vi "Main.vi"() -> ()   [LabVIEW 2017, in "GUI.lvlib"]
doc: "This template is based from the Queued Message Handler design pattern and the Queued Message Handler Project Template that ships with LabVIEW 2014.\n\nThe main difference is that the Queue is private to this module and communication between modules is done via Broadcast and Request events.\n\nRequest events are wrapped via public API methods and are handled in the Event handler loop in this VI.\nAny module can register for Broadcast events sent by this module.\n\nThe Event Handling Loop generates messages based on user interface actions.\n\nThe Message Handling Loop processes messages generated by the Event Handling Loop, or by other messages. The messages are string values, so new messages can be added easily to the Message Cases case structure in the Message Handling Loop. Each message cluster can also provide an optional value for Message Data, which is a variant that can be converted to whatever message-specific data is required.\n_____\nBased on Delacor QMH Project Template 3.1.0.34."
uses:
  GUI.lvlib
  <vilib>/Delacor/Delacor QMH/Libraries/Module Admin_class/Delacor_lib_QMH_Module Admin.lvclass
  Module Buttons--radio button.ctl
  Module Data--cluster.ctl
  Show Panel Argument--cluster.ctl
  Hide Panel Argument--cluster.ctl
  Stop Argument--cluster.ctl
  <vilib>/Delacor/Delacor QMH/Libraries/Module Admin_class/Delacor_lib_QMH_Module Admin.lvclass/Delacor_lib_QMH_Module Admin.ctl
  <vilib>/Delacor/Delacor QMH/Libraries/Module Admin_class/Delacor_lib_QMH_Get External Launch.vi
  <vilib>/Utility/error.llb/Error Cluster From Error Code.vi
  <vilib>/Delacor/Delacor QMH/Libraries/Message Queue_class/Delacor_lib_QMH_Enqueue Message (Single).vi
  <vilib>/ErrorRing/Error Ring.xnode
  <vilib>/Delacor/Delacor QMH/Libraries/Message Queue_class/Delacor_lib_QMH_Message Queue.lvclass
panel:
  in  "Select":T1 caption="Radio Buttons"
  out "Boolean":bool
  in  "Simulate MHL Error":bool
  in  "Simulate EHL Error":bool
  out "error out":errorcluster
  in  "Module Admin":refnum<class "Delacor_lib_QMH_Module Admin.lvclass">
  out "Status":string
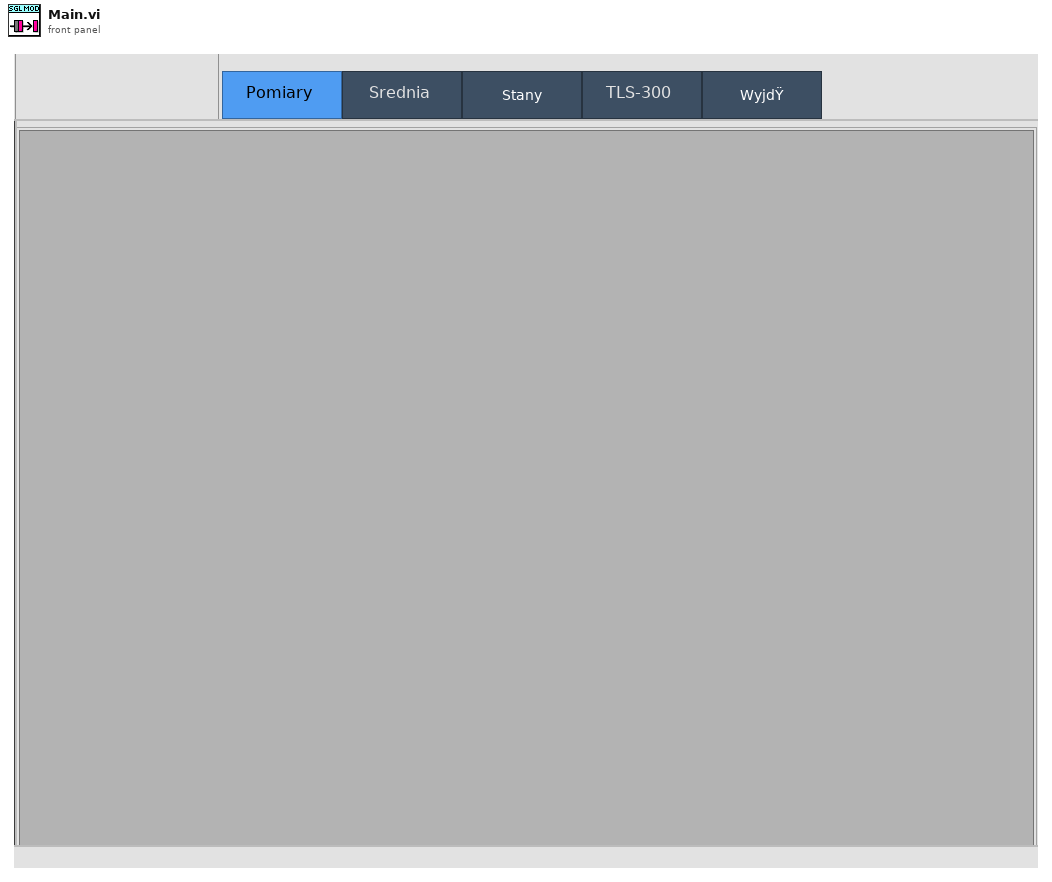
[diagram p1: front panel]
types:
  T1 = typedef "GUI.lvlib/Module Buttons--radio button.ctl" = enum32{"Temperatura", "Srednia", "Stany", "Liczniki", "Exit"}
  T2 = typedef "GUI.lvlib/Request Events--cluster.ctl" = cluster{"Stop Module":refnum<user-event>, "Show Panel":refnum<user-event>, "Hide Panel":refnum<user-event>, "Get Module Execution Status":refnum<user-event>, "Show Diagram":refnum<user-event>}
  T3 = typedef "GUI.lvlib/Module Data--cluster.ctl" = cluster{"Status":string, "subVI Ref.":refnum<vi>[]}
  T4 = typedef "GUI.lvlib/Show Panel Argument--cluster.ctl" = cluster{"Show Panel?":bool}
  T5 = typedef "GUI.lvlib/Hide Panel Argument--cluster.ctl" = cluster{"Hide Panel?":bool}
  T6 = typedef "GUI.lvlib/Stop Argument--cluster.ctl" = cluster{"Origin":string, "Exit via Stop Module Req?":bool, "Wait for Module to stop?":bool}
  T7 = enum32{"Invalid", "Standard", "Closed", "Hidden", "Minimized", "Maximized"}
  T8 = enum32{"invalid lock state", "Not Locked", "Locked (No Password)", "Password-protected"}
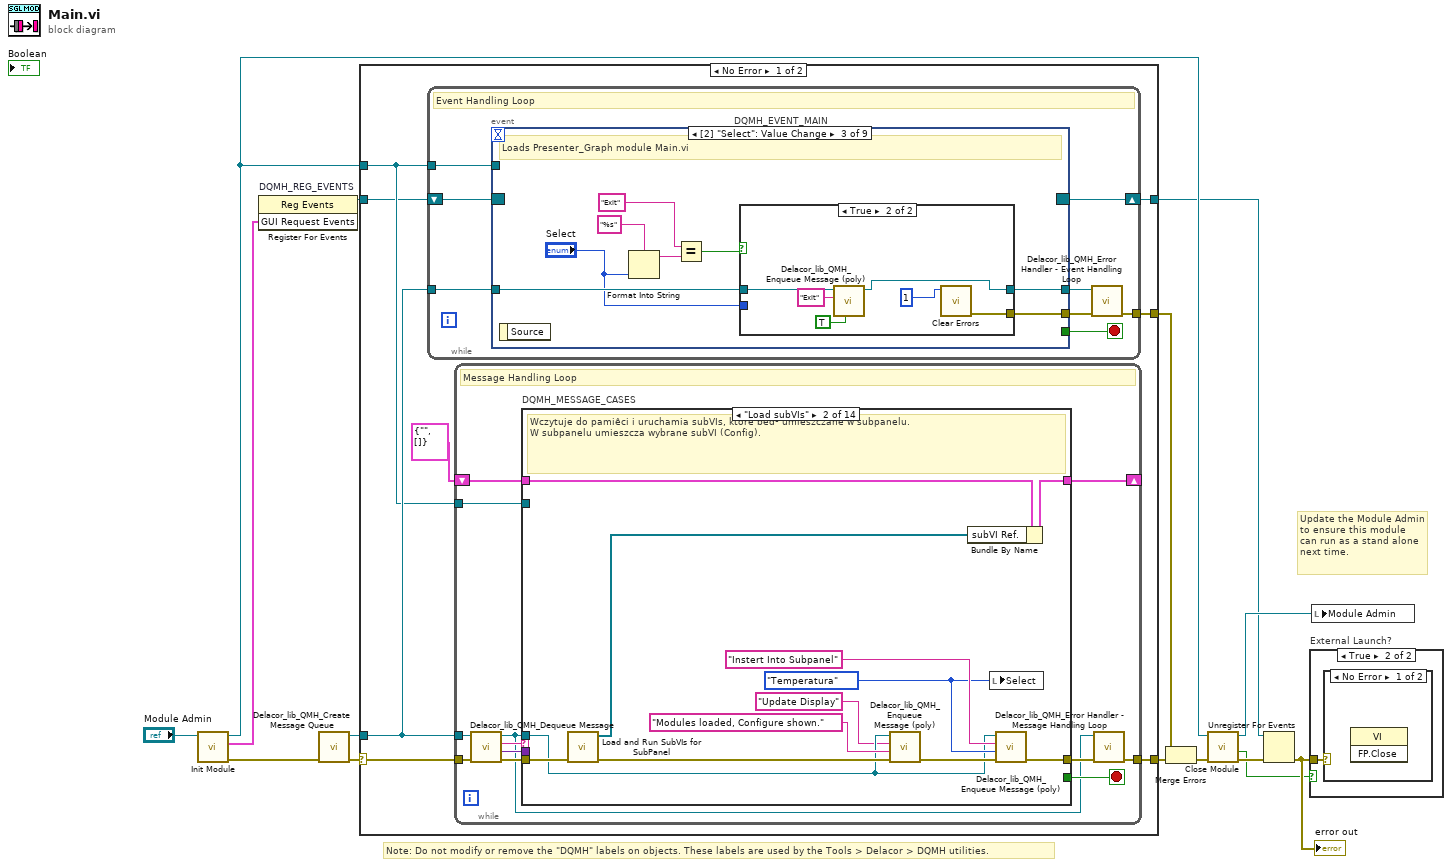
[diagram p0: block diagram]
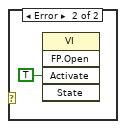
[diagram p3: hidden frame]
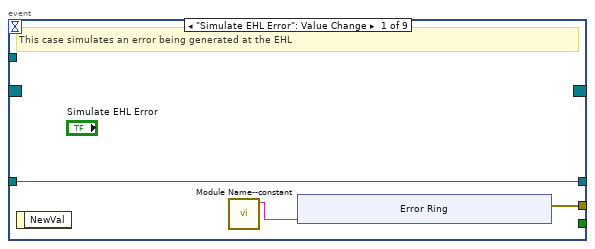
[diagram p4: hidden frame]
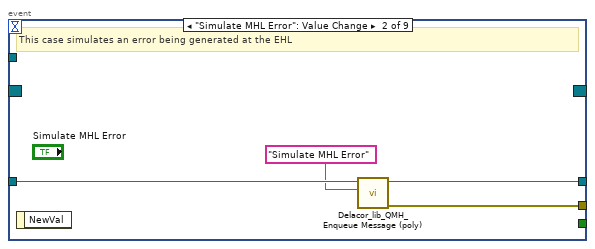
[diagram p5: hidden frame]
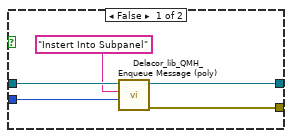
[diagram p6: hidden frame]
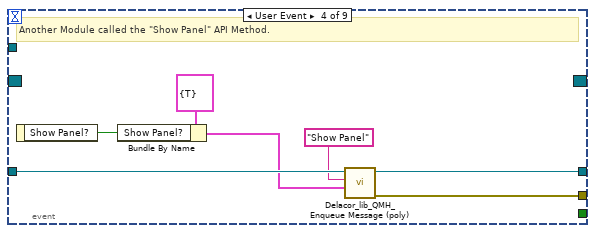
[diagram p7: hidden frame]
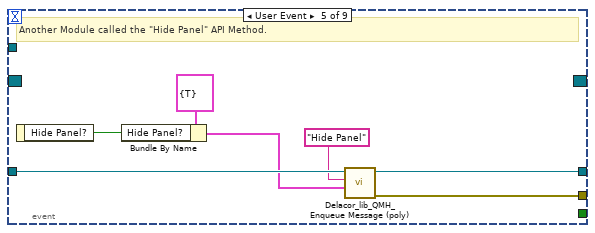
[diagram p8: hidden frame]
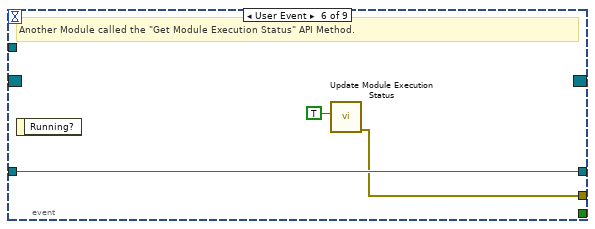
[diagram p9: hidden frame]
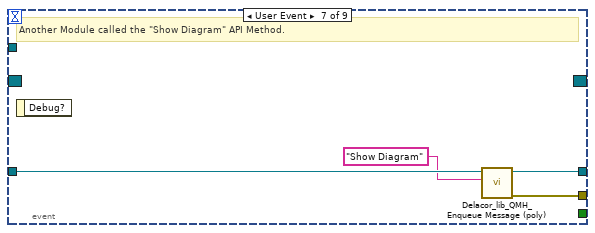
[diagram p10: hidden frame]
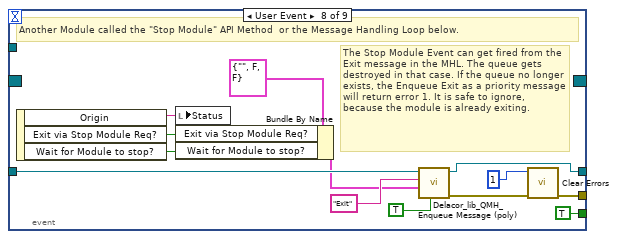
[diagram p11: hidden frame]
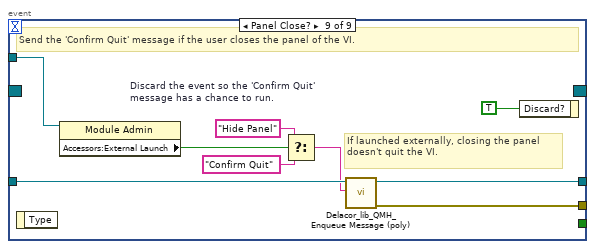
[diagram p12: hidden frame]
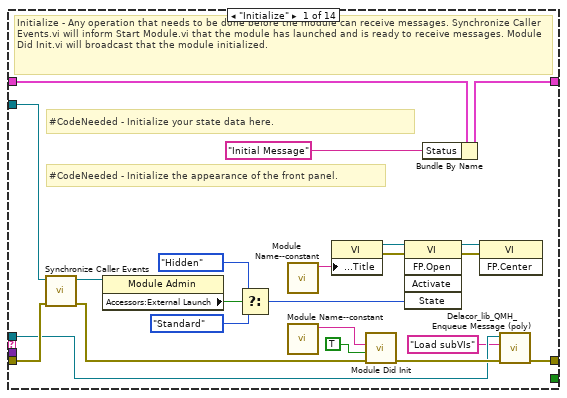
[diagram p13: hidden frame]
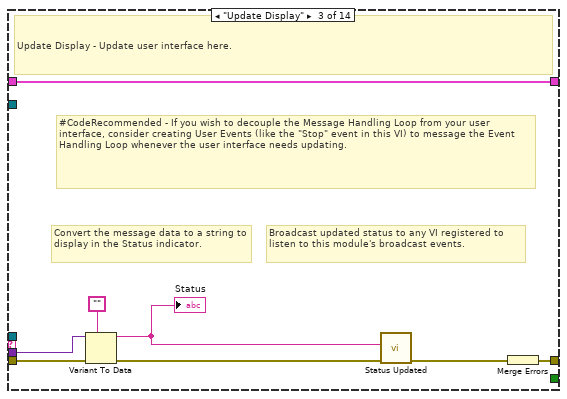
[diagram p14: hidden frame]
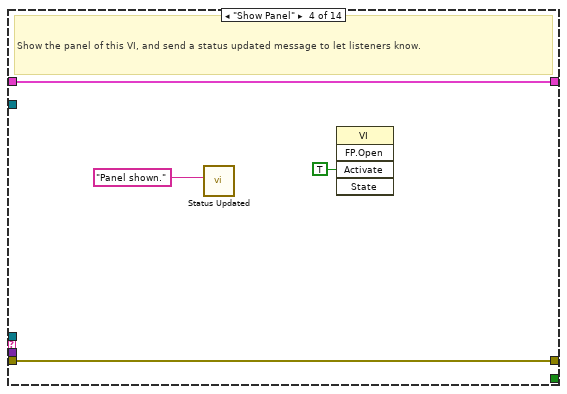
[diagram p15: hidden frame]
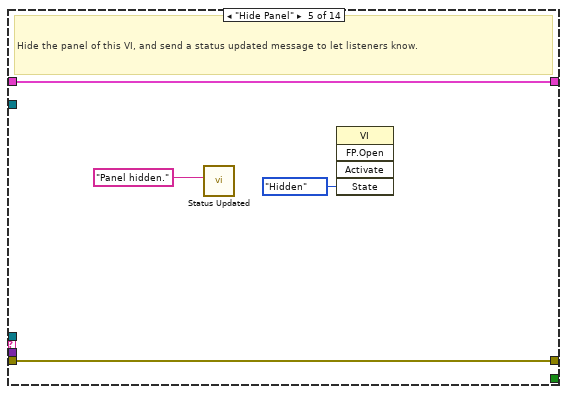
[diagram p16: hidden frame]
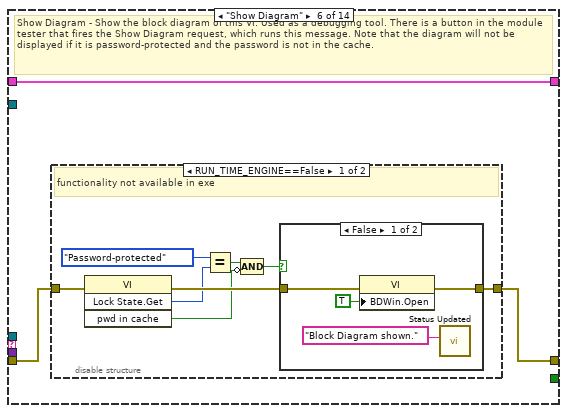
[diagram p17: hidden frame]
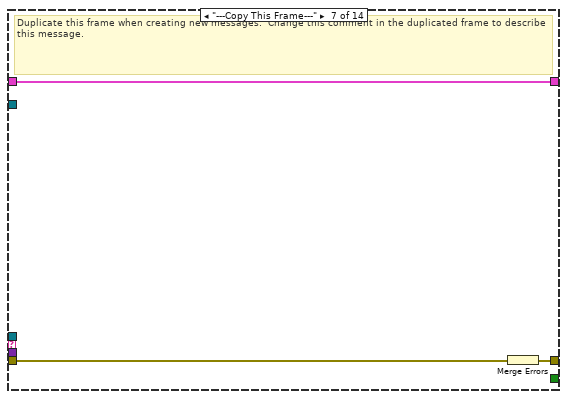
[diagram p20: hidden frame]
diagram:
  # "Note: Do not modify or remove the \"DQMH\" labels on objects. These labels are used by the Tools > Delacor > DQMH utilities."
  # "Update the Module Admin to ensure this module can run as a stand alone next time."
  n1 = call "Init Module.vi"("Singleton Module Admin in"="Module Admin") -> ("error out"=w13:errorcluster, "GUI Request Events"=w11:T2, "Singleton Module Admin out"=w15:refnum<class "Delacor_lib_QMH_Module Admin.lvclass">)  [unwired: 8 in]
  n2 = register-events "DQMH_REG_EVENTS"(w11) -> (reference out=w12:refnum<event-registration>)  [unwired: 2 in, 1 out]
  n3 = call <vilib>:"Delacor_lib_QMH_Create Message Queue.vi"("error in (no error)"=w13) -> ("error out"=w2:errorcluster, "Message Queue"=w10:refnum<class "Delacor_lib_QMH_Message Queue.lvclass">)  [unwired: 9 in]
  n4 = case shown="No Error" w2 {
    selector: w2 -> [w18 w284]
    tunnel: [w23 w284] -> w14
    tunnel: [w22 w289] -> w1
    tunnel: w12 -> [w16 w289]
    tunnel: w10 -> [w20 _]
    tunnel: [w19 _] -> w6
    tunnel: w15 -> [w17 w285]
    frame No Error {
      n5 = while {
        tunnel: w20 -> [w31]
        shift-right: [w29] -> w22
        shift-left: w16 -> [w30]
        tunnel: [w25] -> w19
        tunnel: w17 -> [w24]
        stop <- w27 stop-if-true
        # "Event Handling Loop"
        n6 = event "DQMH_EVENT_MAIN" shown="[2] \"Select\": Value Change" {
          selector: w30 -> [_ _ _ _ _ _ _ _ _]
          dyn-events: [_ _ _ _ _ _ _ _ _] -> w29
          timeout: _ -> [_ _ _ _ _ _ _ _ _]
          tunnel: [_ _ _ _ _ _ _ TRUE ("Discard?") _] -> w27
          tunnel: w31 -> [w34 w45 w53 w71 w78 w81 w85 w96 w106]
          tunnel: [w33 w42 w51 w69 w76 w80 w82 w90 w105] -> w28
          tunnel: [w34 w44 w52 w70 w77 w81 w84 w95 w104] -> w26
          tunnel: w24 -> [_ _ _ _ _ _ _ _ w100]
          event "Simulate EHL Error": Value Change {
            # "This case simulates an error being generated at the EHL"
            n7 = event-data() -> ()  [unwired: 1 in, 1 out]
            n8 = call "Module Name--constant.vi"() -> ("Module Name"=w32:string)  [unwired: 11 in]
            n9 = xnode "Error Ring"("parameter 0"=w32) -> ("error out"=w33:errorcluster)
          }
          event "Simulate MHL Error": Value Change {
            # "This case simulates an error being generated at the EHL"
            n10 = event-data() -> ()  [unwired: 1 in, 1 out]
            n11 = call-poly <vilib>:"Delacor_lib_QMH_Enqueue Message (poly).vi"("Message"="Simulate MHL Error", "Message Queue in"=w45) -> ("error out"=w42:errorcluster, "Message Queue out"=w44:refnum<class "Delacor_lib_QMH_Message Queue.lvclass">)  [unwired: 8 in]
          }
          event Value Change {
            # "Loads Presenter_Graph module Main.vi"
            n12 = event-data() -> ()  [unwired: 1 in, 1 out]
            n13 = Format Into String(format string="%s", "Select") -> (resulting string=w49:string)  [unwired: 2 in, 1 out]
            n14 = Equal?(x="Exit", y=w49) -> (x = y?=w47:bool)
            n15 = case shown="True" w47 {
              tunnel: w53 -> [w58 w61]
              tunnel: [w57 w60] -> w52
              tunnel: [w56 w64] -> w51
              tunnel: "Select" -> [w54 _]
              frame False {
                n16 = call-poly <vilib>:"Delacor_lib_QMH_Enqueue Message (poly).vi"("Message Data"=w54, "Message"="Instert Into Subpanel", "Message Queue in"=w58) -> ("error out"=w56:errorcluster, "Message Queue out"=w57:refnum<class "Delacor_lib_QMH_Message Queue.lvclass">)  [unwired: 7 in]
              }
              frame True {
                n17 = call-poly <vilib>:"Delacor_lib_QMH_Enqueue Message (poly).vi"("Priority Message? (F)"=TRUE, "Message"="Exit", "Message Queue in"=w61) -> ("Message Queue out"=w60:refnum<class "Delacor_lib_QMH_Message Queue.lvclass">)  [unwired: 7 in, 1 out]
                n18 = call <vilib>:"Clear Errors.vi"("specific error code to clear (0: all)"=1) -> ("error out"=w64:errorcluster)  [unwired: 5 in, 1 out]
              }
            }
          }
          event User Event {
            # "Another Module called the \"Show Panel\" API Method."
            n19 = event-data() -> ("Show Panel?"=w67:bool)  [unwired: 1 in]
            n20 = Bundle By Name(cluster=T4 {"Show Panel?"=TRUE} ("Show Panel Argument"), "Show Panel?"=w67) -> (w65:T4)
            n21 = call-poly <vilib>:"Delacor_lib_QMH_Enqueue Message (poly).vi"("Message Data"=w65, "Message"="Show Panel", "Message Queue in"=w71) -> ("error out"=w69:errorcluster, "Message Queue out"=w70:refnum<class "Delacor_lib_QMH_Message Queue.lvclass">)  [unwired: 7 in]
          }
          event User Event {
            # "Another Module called the \"Hide Panel\" API Method."
            n22 = event-data() -> ("Hide Panel?"=w73:bool)  [unwired: 1 in]
            n23 = Bundle By Name(cluster=T5 {"Hide Panel?"=TRUE} ("Hide Panel Argument"), "Hide Panel?"=w73) -> (w72:T5)
            n24 = call-poly <vilib>:"Delacor_lib_QMH_Enqueue Message (poly).vi"("Message Data"=w72, "Message"="Hide Panel", "Message Queue in"=w78) -> ("error out"=w76:errorcluster, "Message Queue out"=w77:refnum<class "Delacor_lib_QMH_Message Queue.lvclass">)  [unwired: 7 in]
          }
          event User Event {
            # "Another Module called the \"Get Module Execution Status\" API Method."
            n25 = event-data() -> ()  [unwired: 1 in, 1 out]
            n26 = call "Update Module Execution Status.vi"("Running?"=TRUE) -> ("error out"=w80:errorcluster)  [unwired: 10 in]
          }
          event User Event {
            # "Another Module called the \"Show Diagram\" API Method."
            n27 = event-data() -> ()  [unwired: 1 in, 1 out]
            n28 = call-poly <vilib>:"Delacor_lib_QMH_Enqueue Message (poly).vi"("Message"="Show Diagram", "Message Queue in"=w85) -> ("error out"=w82:errorcluster, "Message Queue out"=w84:refnum<class "Delacor_lib_QMH_Message Queue.lvclass">)  [unwired: 8 in]
          }
          event User Event {
            # "The Stop Module Event can get fired from the Exit message in the MHL. The queue gets destroyed in that case. If the queue no longer exists, the Enqueue Exit as a priority message will return error 1. It is safe to ignore, because the module is already exiting."
            # "Another Module called the \"Stop Module\" API Method  or the Message Handling Loop below."
            n29 = event-data() -> ("Origin"=w94:string, "Exit via Stop Module Req?"=w88:bool, "Wait for Module to stop?"=w87:bool)  [unwired: 1 in]
            n30 = local write "Status"(w94) -> ()
            n31 = Bundle By Name(cluster=T6 {"Origin"="", "Exit via Stop Module Req?"=FALSE, "Wait for Module to stop?"=FALSE} ("Stop Argument"), "Exit via Stop Module Req?"=w88, "Wait for Module to stop?"=w87) -> (w86:T6)
            n32 = call-poly <vilib>:"Delacor_lib_QMH_Enqueue Message (poly).vi"("Priority Message? (F)"=TRUE, "Message Data"=w86, "Message"="Exit", "Message Queue in"=w96) -> ("error out"=w91:errorcluster, "Message Queue out"=w95:refnum<class "Delacor_lib_QMH_Message Queue.lvclass">)  [unwired: 6 in]
            n33 = call <vilib>:"Clear Errors.vi"("error in (no error)"=w91, "specific error code to clear (0: all)"=1) -> ("error out"=w90:errorcluster)  [unwired: 4 in, 1 out]
          }
          event Panel Close? {
            w107 = TRUE  # Discard the event so the 'Confirm Quit' message has a chance to run.
            # "If launched externally, closing the panel doesn't quit the VI."
            # "Send the 'Confirm Quit' message if the user closes the panel of the VI."
            n34 = event-data() -> ()  [unwired: 1 in, 1 out]
            n35 = property class="Module Admin"(reference=w100) -> ("Accessors:External Launch"=w99:bool)  [unwired: 1 in, 2 out]
            n36 = Select(t="Hide Panel" ("Message"), s=w99, f="Confirm Quit" ("Message")) -> (s? t:f=w101:string)
            n37 = call-poly <vilib>:"Delacor_lib_QMH_Enqueue Message (poly).vi"("Message"=w101, "Message Queue in"=w106) -> ("error out"=w105:errorcluster, "Message Queue out"=w104:refnum<class "Delacor_lib_QMH_Message Queue.lvclass">)  [unwired: 8 in]
            n38 = event-data("Discard?"=w107) -> ()  [unwired: 1 in, 1 out]
          }
        }
        n39 = call-dynamic "Delacor_lib_QMH_Error Handler - Event Handling Loop.vi"("error in (no error)"=w28, "Message Queue in"=w26) -> ("dup error in"=w25:errorcluster)  [unwired: 8 in, 1 out]
      }
      n40 = while {
        tunnel: w20 -> [w111]
        shift-right: [w117] -> _
        shift-left: T3 {"Status"="", "subVI Ref."=[]} ("Data Cluster") -> [w118]
        tunnel: w18 -> [w115]
        tunnel: [w109] -> w23
        tunnel: w17 -> [w108]
        stop <- w116 stop-if-true
        # "Message Handling Loop"
        n41 = call-dynamic "Delacor_lib_QMH_Dequeue Message.vi"("error in (no error)"=w115, "Message Queue in"=w111) -> ("error out"=w114:errorcluster, "Message Data"=w112:variant, "Message"=w113:string, "Message Queue out"=w110:refnum<class "Delacor_lib_QMH_Message Queue.lvclass">)  [unwired: 6 in]
        n42 = case "DQMH_MESSAGE_CASES" shown="\"Load subVIs\"" w113 {
          selector: w113 -> [_ _ _ _ _ _ _ _ _ _ _ _ _ w271]
          tunnel: w110 -> [w121 w143 _ _ _ _ _ w191 _ _ w227 w242 w262 _]
          tunnel: w114 -> [w131 w150 w159 w165 w166 w171 w189 w207 w211 w216 w233 w246 w264 _]
          tunnel: [w122 w148 w160 w165 w166 w170 w187 w208 w209 w214 w224 w244 w259 w272] -> w119
          tunnel: w118 -> [w130 w153 w161 w164 w169 w172 w188 w202 w210 w215 w232 w245 w251 w273]
          tunnel: [w129 w152 w161 w164 w169 w172 w188 w202 w210 w215 w232 w245 w251 w273] -> w117
          tunnel: [_ _ _ _ _ _ _ _ _ _ _ _ w261 _] -> w116
          tunnel: w112 -> [_ _ w158 _ _ _ _ w205 _ _ w231 _ w258 _]
          tunnel: w108 -> [w132 _ _ _ _ _ _ _ _ _ w226 _ w252 _]
          frame "Initialize" {
            # "#CodeNeeded - Initialize the appearance of the front panel."
            # "#CodeNeeded - Initialize your state data here."
            # "Initialize - Any operation that needs to be done before the module can receive messages. Synchronize Caller Events.vi will inform Start Module.vi that the module has launched and is ready to receive messages. Module Did Init.vi will broadcast that the module initialized."
            n43 = call "Synchronize Caller Events.vi"("error in (no error)"=w131, "Singleton Module Admin in"=w132) -> ("error out"=w125:errorcluster, "Singleton Module Admin out"=w124:refnum<class "Delacor_lib_QMH_Module Admin.lvclass">)  [unwired: 8 in]
            n44 = property class="Module Admin"(reference=w124) -> ("Accessors:External Launch"=w136:bool)  [unwired: 1 in, 2 out]
            n45 = Select(t=T7."Hidden" ("State"), s=w136, f=T7."Standard" ("State")) -> (s? t:f=w133:T7)
            n46 = call "Module Name--constant.vi"() -> ("Module Name"=w141:string)  [unwired: 11 in]
            n47 = call "Module Name--constant.vi"() -> ("Module Name"=w126:string)  [unwired: 11 in]
            n48 = property class="VI"("Front Panel.Title"=w141) -> (reference out=w139:refnum<vi>, error out=w140:errorcluster)  [unwired: 2 in]
            n49 = call "Module Did Init.vi"("error in (no error)"=w125, "Initialized?"=TRUE, "Origin"=w126) -> ("error out"=w123:errorcluster)  [unwired: 8 in]
            n50 = invoke class="VI" method="FP.Open"(reference=w139, error in=w140, "State"=w133) -> (reference out=w138:refnum<vi>, error out=w137:errorcluster)  [unwired: 2 in, 3 out]
            n51 = Bundle By Name(cluster=w130, "Status"="Initial Message" ("Initial Message")) -> (w129:T3)
            n52 = invoke class="VI" method="FP.Center"(reference=w138, error in=w137) -> ()  [unwired: 1 in, 3 out]
            n53 = call-poly <vilib>:"Delacor_lib_QMH_Enqueue Message (poly).vi"("error in (no error)"=w123, "Message"="Load subVIs", "Message Queue in"=w121) -> ("error out"=w122:errorcluster)  [unwired: 7 in, 1 out]
          }
          frame "Load subVIs" {
            w147 = Module_Buttons--radio_button."Temperatura" ("Select")
            # "Wczytuje do pamiêci i uruchamia subVIs, które bêd¹ umieszczane w subpanelu.\nW subpanelu umieszcza wybrane subVI (Config)."
            n54 = call "Load and Run SubVIs for SubPanel.vi"("error in (no error)"=w150) -> ("error out"=w146:errorcluster, "subVIs Ref."=w151:refnum<vi>[])  [unwired: 9 in]
            n55 = call-poly <vilib>:"Delacor_lib_QMH_Enqueue Message (poly).vi"("error in (no error)"=w146, "Message Data"="Modules loaded, Configure shown." ("Message"), "Message"="Update Display", "Message Queue in"=w143) -> ("error out"=w145:errorcluster)  [unwired: 6 in, 1 out]
            n56 = Bundle By Name(cluster=w153, "subVI Ref."=w151) -> (w152:T3)
            n57 = local write "Select"(w147) -> ()
            n58 = call-poly <vilib>:"Delacor_lib_QMH_Enqueue Message (poly).vi"("error in (no error)"=w145, "Message Data"=w147, "Message"="Instert Into Subpanel", "Message Queue in"=w143) -> ("error out"=w148:errorcluster)  [unwired: 6 in, 1 out]
          }
          frame "Update Display" {
            # "Broadcast updated status to any VI registered to listen to this module's broadcast events."
            # "Convert the message data to a string to display in the Status indicator."
            # "#CodeRecommended - If you wish to decouple the Message Handling Loop from your user interface, consider creating User Events (like the \"Stop\" event in this VI) to message the Event Handling Loop whenever the user interface needs updating."
            # "Update Display - Update user interface here."
            n59 = Variant To Data(error in=w159, type="", Variant=w158) -> (data=w156:string, error out=w155:errorcluster)
            "Status" <- w156
            n60 = call "Status Updated.vi"("error in (no error)"=w155, "Status"=w156) -> ("error out"=w154:errorcluster)  [unwired: 9 in]
            n61 = Merge Errors(w154) -> (w160:errorcluster)
          }
          frame "Show Panel" {
            # "Show the panel of this VI, and send a status updated message to let listeners know."
            n62 = call "Status Updated.vi"("Status"="Panel shown." ("format string")) -> ()  [unwired: 10 in, 1 out]
            n63 = invoke class="VI" method="FP.Open"("Activate"=TRUE ("Activate?")) -> ()  [unwired: 4 in, 5 out]
          }
          frame "Hide Panel" {
            # "Hide the panel of this VI, and send a status updated message to let listeners know."
            n64 = call "Status Updated.vi"("Status"="Panel hidden." ("format string")) -> ()  [unwired: 10 in, 1 out]
            n65 = invoke class="VI" method="FP.Open"("State"=T7."Hidden") -> ()  [unwired: 4 in, 5 out]
          }
          frame "Show Diagram" {
            # "Show Diagram - Show the block diagram of this VI. Used as a debugging tool. There is a button in the module tester that fires the Show Diagram request, which runs this message. Note that the diagram will not be displayed if it is password-protected and the password is not in the cache."
            n66 = disable-structure shown="RUN_TIME_ENGINE==False" {
              disable-tunnel: [w180 w186] -> w170
              disable-tunnel: w171 -> [w179 w186]
              frame condition #0 (active) {
                # "functionality not available in exe"
                n67 = invoke class="VI" method="Lock State.Get"(error in=w179) -> (error out=w178:errorcluster, "Get Lock State"=w177:T8, "pwd in cache"=w174:bool)  [unwired: 3 in, 1 out]
                n68 = Equal?(x=T8."Password-protected", y=w177) -> (x = y?=w175:bool)
                n69 = Compound Arithmetic op=AND(w175, invert w174) -> (w173:bool)
                n70 = case shown="False" w173 {
                  tunnel: [w183 w185] -> w180
                  tunnel: w178 -> [w181 w185]
                  frame False {
                    n71 = property class="VI"(error in=w181, "BDWin.Open"=TRUE ("Block Diagram Window:Open")) -> (error out=w183:errorcluster)  [unwired: 1 in, 1 out]
                    n72 = call "Status Updated.vi"("Status"="Block Diagram shown." ("format string")) -> ()  [unwired: 10 in, 1 out]
                  }
                  frame True {
                    # "Password-protected VI, and the password is not in the cache. Do not show the diagram."
                  }
                }
              }
              frame condition #1 {
              }
            }
          }
          frame "---Copy This Frame---" {
            # "Duplicate this frame when creating new messages.  Change this comment in the duplicated frame to describe this message."
            n73 = Merge Errors(w189) -> (w187:errorcluster)
          }
          frame "Instert Into Subpanel" {
            # "Instert VI into subpanel"
            n74 = Unbundle By Name(w202) -> ("subVI Ref."=w201:refnum<vi>[])
            n75 = Variant To Data(error in=w207, type=Module_Buttons--radio_button."Temperatura" ("Select"), Variant=w205) -> (data=w200:T1, error out=w204:errorcluster)
            n76 = Index Array(array=w201, index=w200) -> (element=w199:refnum<vi>)
            n77 = invoke on="Sub Panel" class="SubPnl" method="Remove VI"(error in=w204) -> (error out=w203:errorcluster)  [unwired: 2 in, 2 out]
            n78 = invoke on="Sub Panel" class="SubPnl" method="Insert VI"(error in=w203, "VI Ref"=w199) -> (error out=w206:errorcluster)  [unwired: 2 in, 3 out]
            n79 = property class="VI"(reference=w199) -> ("Name"=w195:string, "Front Panel.Title"=w190:string)  [unwired: 1 in, 2 out]
            n80 = Concatenate Strings(w190, " loaded" ("string")) -> (w193:string)
            n81 = call "Subpanel VI Loaded.vi"("error in (no error)"=w206, "VI Name"=w195) -> ("error out"=w197:errorcluster)  [unwired: 9 in]
            n82 = call-poly <vilib>:"Delacor_lib_QMH_Enqueue Message (poly).vi"("error in (no error)"=w197, "Message Data"=w193, "Message"="Update Display", "Message Queue in"=w191) -> ("error out"=w196:errorcluster)  [unwired: 6 in, 1 out]
            n83 = Merge Errors(w196) -> (w208:errorcluster)
          }
          frame "--- Exit and Error Handling---" {
            # "Separator - The following cases handle errors and exit messages."
            n84 = Merge Errors(w211) -> (w209:errorcluster)
          }
          frame "Simulate MHL Error" {
            # "Simulate an error occurring at the MHL"
            n85 = call "Module Name--constant.vi"() -> ("Module Name"=w213:string)  [unwired: 11 in]
            n86 = xnode "Error Ring"("parameter 0"=w213) -> ("error out"=w212:errorcluster)
            n87 = Merge Errors(w216, w212) -> (w214:errorcluster)
          }
          frame "Error" {
            # "#CodeRecommended - If you ever change the name of this \"Error\" message, you'll need to update the name in the Check Loop Error.vi as well."
            # "#CodeRecommended - If the module is running in standalone mode (External Launch = FALSE), this code will pop up an error dialog and call the 'Exit' message if an error occurs. Add more fine-grained error handling here."
            # "Error - Check the error message data and respond accordingly. This message is sent by the \"Error Handler\" VIs at the end of each loop in this application."
            n88 = property class="Module Admin"(reference=w226) -> ("Accessors:External Launch"=w225:bool)  [unwired: 1 in, 2 out]
            n89 = Variant To Data(error in=w233, type=errorcluster {"status"=FALSE, "code"=0, "source"=""} ("error constant"), Variant=w231) -> (data=w234:errorcluster, error out=w229:errorcluster)
            n90 = call "Error Reported.vi"("Error"=w234) -> ()  [unwired: 10 in, 1 out]
            n91 = case shown="False" w225 {
              tunnel: [w239 _] -> w228
              tunnel: w227 -> [w238 _]
              tunnel: w234 -> [w235 _]
              frame False {
                # "If the module is running standalone, then pop up an error dialog and call the \"Exit\" message."
                n92 = call <vilib>:"Simple Error Handler.vi"("error in (no error)"=w235) -> ()  [unwired: 4 in, 5 out]
                n93 = call-poly <vilib>:"Delacor_lib_QMH_Enqueue Message (poly).vi"("Priority Message? (F)"=TRUE, "Message"="Exit", "Message Queue in"=w238) -> ("error out"=w239:errorcluster)  [unwired: 7 in, 1 out]
              }
              frame True {
                # "If the module was launched externally, calling the Error Reported broadcast VI is the only action performed by the \"Error\" message. The module's caller can then process the error appropriately."
              }
            }
            n94 = Merge Errors(w229, w228) -> (w224:errorcluster)
            n95 = local write "error out"(w224) -> ()
          }
          frame "Confirm Quit" {
            # "#CodeNeeded - If you want to provide an \"Are you sure\" dialog (or some other notification) before the application exits, place that code here. This message is typically sent from a Panel Close? event."
            # "Confirm Quit - Message that can confirm whether or not the user wants to exit the application."
            n96 = call-poly <vilib>:"Delacor_lib_QMH_Enqueue Message (poly).vi"("Priority Message? (F)"=TRUE, "error in (no error)"=w246, "Message"="Exit", "Message Queue in"=w242) -> ("error out"=w243:errorcluster)  [unwired: 6 in, 1 out]
            n97 = Merge Errors(w243) -> (w244:errorcluster)
          }
          frame "Exit" {
            w256 = 91  # 91: not all Exit messages will have an argument
            w261 = TRUE  # Stop the VI
            # "Release the message queue reference"
            # "Exit - Exit the application."
            n98 = control-ref of="This VI"() -> (w253:refnum<vi>)
            n99 = Variant To Data(error in=w264, type=T6 {"Origin"="", "Exit via Stop Module Req?"=FALSE, "Wait for Module to stop?"=FALSE} ("Stop Argument"), Variant=w258) -> (data=w254:T6, error out=w257:errorcluster)
            n100 = call "Handle Exit.vi"("Stop Argument"=w254, "Admin in"=w252, "VI reference"=w253) -> ("error out"=w250:errorcluster)  [unwired: 7 in, 1 out]
            n101 = call <vilib>:"Clear Errors.vi"("error in (no error)"=w257, "specific error code to clear (0: all)"=w256) -> ("error out"=w263:errorcluster)  [unwired: 4 in, 1 out]
            n102 = Unbundle By Name(w251) -> ("subVI Ref."=w247:refnum<vi>[])
            n103 = invoke on="Sub Panel" class="SubPnl" method="Remove VI"(error in=w250) -> (error out=w248:errorcluster)  [unwired: 2 in, 2 out]
            n104 = for {
              shift-right: [w269] -> w249
              shift-left: w248 -> [w268]
              tunnel: w247 -> [w265] mode=indexing
              n105 = invoke class="VI" method="Abort VI"(reference=w265, error in=w268) -> (reference out=w266:refnum<vi>, error out=w267:errorcluster)  [unwired: 1 in, 1 out]
              n106 = Close Reference(reference=w266, error in (no error)=w267) -> (error out=w269:errorcluster)
            }
            n107 = call-dynamic "Delacor_lib_QMH_Release Message Queue.vi"("error in (no error)"=w263, "Message Queue"=w262) -> ("error out"=w260:errorcluster)  [unwired: 9 in]
            n108 = Merge Errors(w249, w260) -> (w259:errorcluster)
          }
          frame Default {
            # "'Default' case only runs if there is a message that isn't defined in any of the other cases.  Output a programming error."
            n109 = call "Module Name--constant.vi"() -> ("Module Name"=w270:string)  [unwired: 11 in]
            n110 = xnode "Error Ring"("parameter 0"=w271, "parameter 1"=w270) -> ("error out"=w272:errorcluster)
          }
        }
        n111 = call-dynamic "Delacor_lib_QMH_Error Handler - Message Handling Loop.vi"("error in (no error)"=w119, "Message Queue in"=w110) -> ("dup error in"=w109:errorcluster)  [unwired: 8 in, 1 out]
      }
    }
    frame Error {
      # "Synchronize Caller Events.vi will inform Start Module.vi that the module has launched and will let the code calling Start Module.vi register for broadcasts and would permit the caller receive the broadcast that an error occurred at launch time."
      n112 = call "Synchronize Caller Events.vi"("Singleton Module Admin in"=w285) -> ("error out"=w282:errorcluster)  [unwired: 9 in, 1 out]
      n113 = call "Module Name--constant.vi"() -> ("Module Name"=w288:string)  [unwired: 11 in]
      n114 = Format Into String(format string="An error occurred during initialization. %s is no longer running.", w288) -> (resulting string=w286:string)  [unwired: 2 in, 1 out]
      n115 = Merge Errors(w284, w282) -> (w283:errorcluster)
      n116 = call "Error Reported.vi"("Additional Information"=w286, "Error"=w283) -> ()  [unwired: 9 in, 1 out]
    }
  }
  n117 = Merge Errors(w6, w14) -> (w5:errorcluster)
  n118 = call "Close Module.vi"("error in (no error)"=w5, "Module Admin in"=w15) -> ("error out"=w8:errorcluster, "External Launch"=w3:bool, "Module Admin out"=w7:refnum<class "Delacor_lib_QMH_Module Admin.lvclass">)  [unwired: 7 in]
  n119 = Unregister For Events(event registration refnum=w1, error in=w8) -> (error out=w4:errorcluster)
  "error out" <- w4
  n120 = case "External Launch?" shown="True" w3 {
    tunnel: w4 -> [_ w290]
    frame False {
    }
    frame True {
      n121 = case shown="No Error" w290 {
        frame No Error {
          n122 = invoke class="VI" method="FP.Close"() -> ()  [unwired: 3 in, 3 out]
        }
        frame Error {
          n123 = invoke class="VI" method="FP.Open"("Activate"=TRUE ("Activate?")) -> ()  [unwired: 4 in, 5 out]
        }
      }
    }
  }
  n124 = local write "Module Admin"(w7) -> ()
